vi "SetCtrlPropGen.vi"(4 "Error in":errorcluster, 6 "Énum":T1(ring), 7 "Controls":refnum<vi>[](array[refnum])) -> (0 "Error out":errorcluster, 3 "Controls Out":refnum<vi>[](array[refnum]))   [LabVIEW 2012]
doc: "Ce VI ouvre le fichier de sauvegarde des modèles et lit les positions du modèle spécifié."
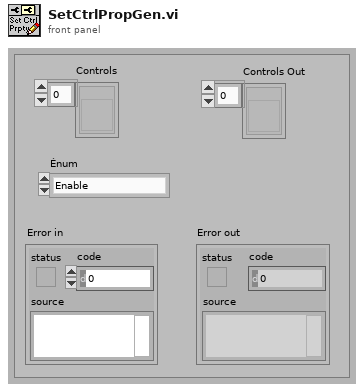
[diagram p1: front panel]
types:
  T1 = enum16{"Enable", "Disable", "DisAndGrayed", "ReinitToDefVal", "EnumElementsArr"}
  T2 = enum8{"Enabled", "Disabled", "Disabled and Grayed Out"}
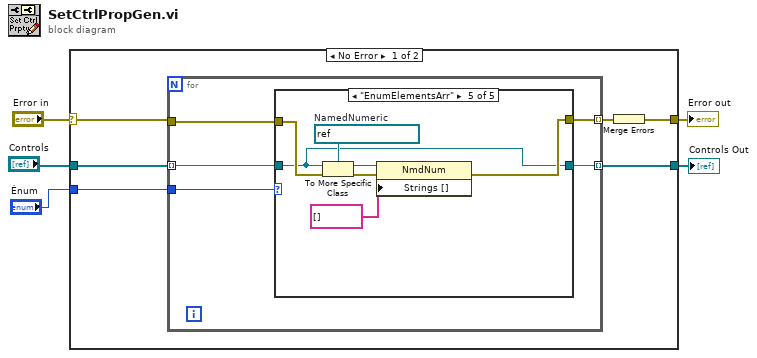
[diagram p0: block diagram]
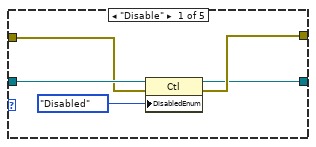
[diagram p2: hidden frame]
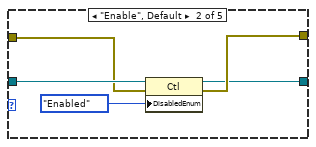
[diagram p3: hidden frame]
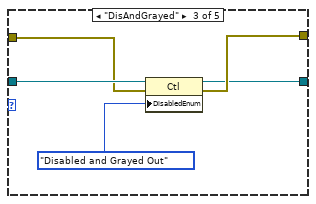
[diagram p4: hidden frame]
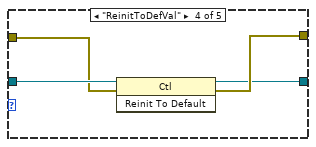
[diagram p5: hidden frame]
diagram:
  n1 = case shown="No Error" "Error in" {
    selector: "Error in" -> [w11 w43]
    tunnel: [w9 w43] -> w5
    tunnel: [w8 w42] -> w3
    tunnel: "Controls" -> [w7 w42]
    tunnel: "Énum" -> [w6 _]
    frame No Error {
      n2 = for {
        tunnel: w7 -> [w16] mode=indexing
        tunnel: w11 -> [w15]
        tunnel: [w14] -> w10 mode=indexing
        tunnel: [w13] -> w8 mode=indexing
        tunnel: w6 -> [w12]
        n3 = case shown="\"EnumElementsArr\"" w12 {
          tunnel: w16 -> [w21 w26 w31 w35 w36]
          tunnel: w15 -> [w19 w24 w29 w34 w41]
          tunnel: [w18 w23 w28 w33 w40] -> w14
          tunnel: [w17 w22 w27 w32 w36] -> w13
          frame "Disable" {
            n4 = property class="Ctl"(reference=w21, error in=w19, "DisabledEnum"=T2."Disabled" ("Désactivé")) -> (reference out=w17:refnum<vi>, error out=w18:errorcluster)
          }
          frame "Enable", Default {
            n5 = property class="Ctl"(reference=w26, error in=w24, "DisabledEnum"=T2."Enabled" ("Désactivé")) -> (reference out=w22:refnum<vi>, error out=w23:errorcluster)
          }
          frame "DisAndGrayed" {
            n6 = property class="Ctl"(reference=w31, error in=w29, "DisabledEnum"=T2."Disabled and Grayed Out" ("Désactivé")) -> (reference out=w27:refnum<vi>, error out=w28:errorcluster)
          }
          frame "ReinitToDefVal" {
            n7 = invoke class="Ctl" method="Reinit To Default"(reference=w35, error in=w34) -> (reference out=w32:refnum<vi>, error out=w33:errorcluster)  [unwired: 1 in, 1 out]
          }
          frame "EnumElementsArr" {
            w38 = refnum<vi> refnum  # NamedNumeric
            n8 = To More Specific Class(target class=w38, reference=w36) -> (specific class reference=w39:refnum<vi>)  [unwired: 1 in, 1 out]
            n9 = property class="NmdNum"(reference=w39, error in=w41, "Strings []"=string[] [] ("Noms d'éléments")) -> (error out=w40:errorcluster)  [unwired: 1 out]
          }
        }
      }
      n10 = Merge Errors(w10) -> (w9:errorcluster)
    }
    frame Error {
    }
  }
  "Error out" <- w5
  "Controls Out" <- w3
